vi "Render.vi"(7 "Renderer":refnum<class "Renderer.lvclass">, 10 "Camera":refnum<class "Camera.lvclass">, 11 "Thrust Dot in":refnum<class "Thrust Dot.lvclass">) -> ()   [LabVIEW 2021, in "Thrust Dot.lvclass"]
uses:
  Thrust Dot.lvclass
  Camera/Camera.lvclass
  Renderer/Renderer.lvclass
  Thrust Dot.lvclass/Thrust Dot.ctl
  Vector 2D/Vector 2D.lvclass/Vector 2D.ctl
  LabSDL2/Source/Libraries/LibSDL2 Wrapper/LibSDL2.lvlib
  Vector 2D/Vector 2D.lvclass
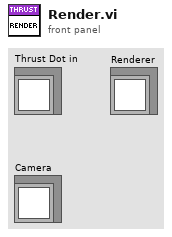
[diagram p1: front panel]
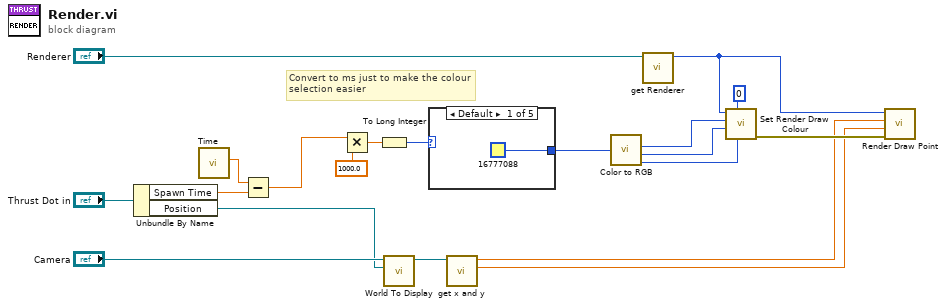
[diagram p0: block diagram]
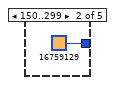
[diagram p2: hidden frame]
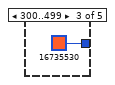
[diagram p3: hidden frame]
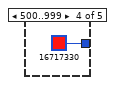
[diagram p4: hidden frame]
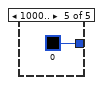
[diagram p5: hidden frame]
diagram:
  # "Convert to ms just to make the colour selection easier"
  n1 = Unbundle By Name("Thrust Dot in") -> ("Spawn Time"=w19:sgl, "Position"=w5:refnum<class "Vector 2D.lvclass">)
  n2 = call "Time.vi"() -> ("Time [s]"=w1:sgl)  [unwired: 10 in, 1 out]
  n3 = Subtract(x=w1, y=w19) -> (x-y=w14:sgl)
  n4 = Multiply(x=w14, y=1000.0) -> (x*y=w12:dbl)
  n5 = To Long Integer(number=w12) -> (32bit integer=w11:i32)
  n6 = call "World To Display.vi"("World Position"=w5, "Camera in"="Camera") -> ("Display Position"=w4:refnum<class "Vector 2D.lvclass">)  [unwired: 9 in]
  n7 = case shown="Default" w11 {
    tunnel: [u32 16777088 ("Color") u32 16759129 ("Color") u32 16735530 ("Color") u32 16717330 ("Color") u32 0 ("Color")] -> w10
    frame Default {
    }
    frame 150..299 {
    }
    frame 300..499 {
    }
    frame 500..999 {
    }
    frame 1000.. {
    }
  }
  n8 = call "get x and y.vi"("Vector 2D in"=w4) -> ("y"=w2:sgl, "x"=w3:sgl)  [unwired: 9 in]
  n9 = call <vilib>:"Color to RGB.vi"("Color"=w10) -> ("R"=w15:u8, "G"=w16:u8, "B"=w17:u8)  [unwired: 1 out]
  n10 = call-dynamic "get Renderer.vi"("Renderer in"="Renderer") -> ("Renderer"=w6:u32)  [unwired: 10 in]
  n11 = call "Set Render Draw Colour.vi"("B"=w17, "A"=u8 0, "G"=w16, "R"=w15, "Renderer Pointer"=w6) -> ("error out"=w18:errorcluster)  [unwired: 5 in, 1 out]
  n12 = call "Render Draw Point.vi"("error in"=w18, "y"=w2, "x"=w3, "Renderer Pointer"=w6) -> ()  [unwired: 6 in, 2 out]
